vi "Session_Data.vi"(10 "Session":i32) -> (2 "output cluster":T1)   [LabVIEW 2010]
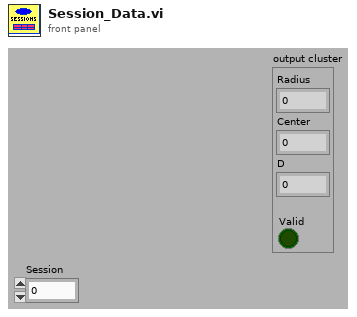
[diagram p1: front panel]
types:
  T1 = cluster{"Radius":dbl, "Center":dbl, "D":dbl, "Valid":bool}
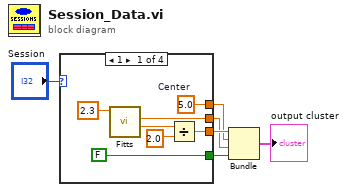
[diagram p0: block diagram]
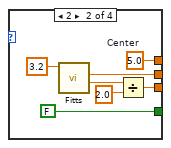
[diagram p2: hidden frame]
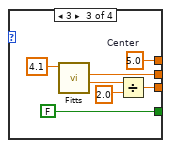
[diagram p3: hidden frame]
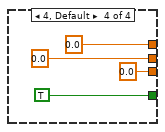
[diagram p4: hidden frame]
diagram:
  n1 = case shown="1" "Session" {
    tunnel: [w10 w15 w21 0.0 ("Radius")] -> w5
    tunnel: [w13 w20 w27 0.0 ("x0")] -> w4
    tunnel: [w7 w14 w23 0.0 ("x0")] -> w3
    tunnel: [FALSE FALSE FALSE TRUE] -> w2
    frame 1 {
      w13 = 5.0  # Center
      n2 = call "Fitts.vi"("ID"=2.3) -> ("W"=w8:dbl, "D"=w7:dbl)  [unwired: 9 in]
      n3 = Divide(x=w8, y=2.0) -> (x/y=w10:dbl)
    }
    frame 2 {
      w20 = 5.0  # Center
      n4 = call "Fitts.vi"("ID"=3.2) -> ("W"=w16:dbl, "D"=w14:dbl)  [unwired: 9 in]
      n5 = Divide(x=w16, y=2.0) -> (x/y=w15:dbl)
    }
    frame 3 {
      w27 = 5.0  # Center
      n6 = call "Fitts.vi"("ID"=4.1) -> ("W"=w22:dbl, "D"=w23:dbl)  [unwired: 9 in]
      n7 = Divide(x=w22, y=2.0) -> (x/y=w21:dbl)
    }
    frame 4, Default {
    }
  }
  n8 = Bundle("Radius"=w5, "x0"=w4, "x0"=w3, w2) -> (→"output cluster":cluster{"Radius":dbl, "x0":dbl, "x0":dbl, bool})  [unwired: 1 in]
